vi "iterate_current_block_offset.vi"(8 "error in (no error)":errorcluster, 11 "GenericWriteSignals in":refnum<class "GenericSignalWriter.lvclass">) -> (0 "error out":errorcluster, 2 "finished?":bool, 3 "GenericWriteSignals out":refnum<class "GenericSignalWriter.lvclass">)   [LabVIEW 2010, in "GenericSignalWriter.lvclass"]
uses:
  GenericSignalWriter.lvclass
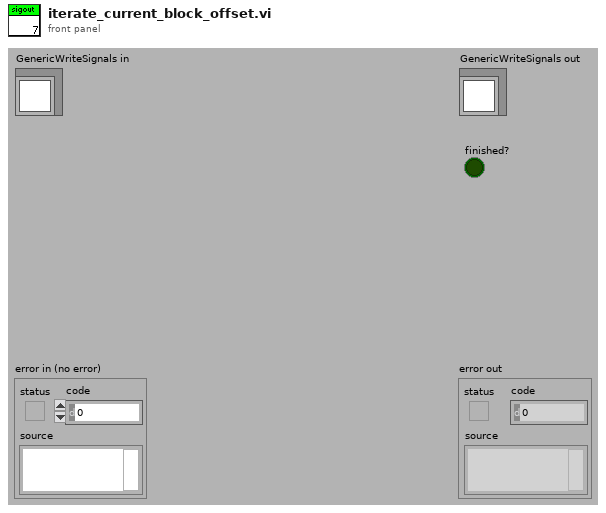
[diagram p1: front panel]
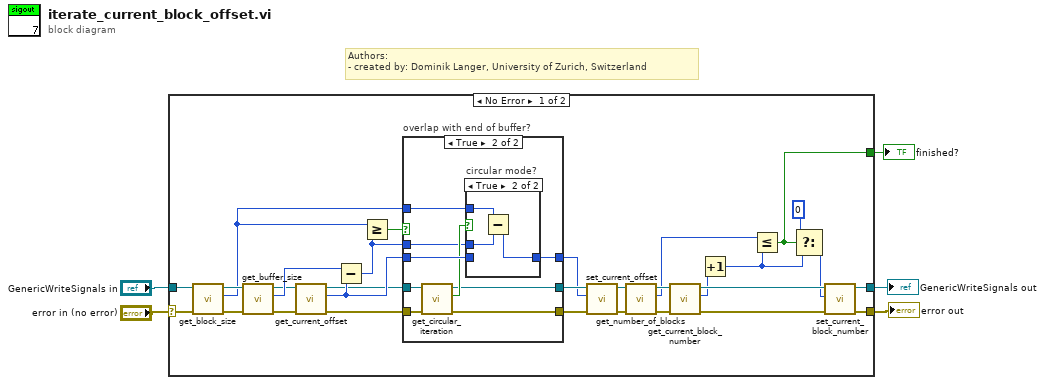
[diagram p0: block diagram]
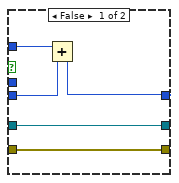
[diagram p2: hidden frame]
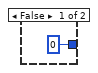
[diagram p3: hidden frame]
diagram:
  # "Authors: \n- created by: Dominik Langer, University of Zurich, Switzerland"
  n1 = case shown="No Error" "error in (no error)" {
    selector: "error in (no error)" -> [w27 w55]
    tunnel: [w18 w55] -> w4
    tunnel: [w19 w54] -> w2
    tunnel: "GenericWriteSignals in" -> [w26 w54]
    tunnel: [w10 _] -> w1
    frame No Error {
      n2 = call "get_block_size.vi"("error in (no error)"=w27, "GenericWriteSignals.lvclass in"=w26) -> ("error out"=w33:errorcluster, "block size"=w29:i32, "GenericWriteSignals.lvclass out"=w32:refnum<class "GenericSignalWriter.lvclass">)  [unwired: 7 out]
      n3 = call-dynamic "get_buffer_size.vi"("error in (no error)"=w33, "GenericWriteSignals.lvclass in"=w32) -> ("error out"=w34:errorcluster, "buffer size (samples)"=w35:i32, "GenericWriteSignals.lvclass out"=w31:refnum<class "GenericSignalWriter.lvclass">)  [unwired: 7 out]
      n4 = call-dynamic "get_current_offset.vi"("error in (no error)"=w34, "GenericWriteSignals.lvclass in"=w31) -> ("error out"=w25:errorcluster, "current offset (samples)"=w28:i32, "GenericWriteSignals.lvclass out"=w24:refnum<class "GenericSignalWriter.lvclass">)  [unwired: 7 out]
      n5 = Subtract(x=w35, y=w28) -> (x-y=w21:i32)
      n6 = Greater Or Equal?(x=w29, y=w21) -> (x >= y?=w30:bool)
      n7 = case "overlap with end of buffer?" shown="True" w30 {
        tunnel: w29 -> [w38 w49]
        tunnel: [w36 w47] -> w20
        tunnel: w28 -> [w37 w48]
        tunnel: w25 -> [w39 w46]
        tunnel: w24 -> [w40 w45]
        tunnel: [w39 w43] -> w23
        tunnel: [w40 w42] -> w22
        tunnel: w21 -> [_ w41]
        frame False {
          n8 = Add(x=w38, y=w37) -> (x+y=w36:i32)
        }
        frame True {
          n9 = call-dynamic "get_circular_iteration.vi"("error in (no error)"=w46, "GenericWriteSignals.lvclass in"=w45) -> ("error out"=w43:errorcluster, "circular iteration?"=w44:bool, "GenericWriteSignals.lvclass out"=w42:refnum<class "GenericSignalWriter.lvclass">)  [unwired: 7 out]
          n10 = case "circular mode?" shown="True" w44 {
            tunnel: w49 -> [_ w53]
            tunnel: w48 -> [_ _]
            tunnel: [0 w51] -> w47
            tunnel: w41 -> [_ w52]
            frame False {
            }
            frame True {
              n11 = Subtract(x=w53, y=w52) -> (x-y=w51:i32)
            }
          }
        }
      }
      n12 = call-dynamic "set_current_offset.vi"("error in (no error)"=w23, "current offset (samples)"=w20, "GenericWriteSignals.lvclass in"=w22) -> ("error out"=w15:errorcluster, "GenericWriteSignals.lvclass out"=w14:refnum<class "GenericSignalWriter.lvclass">)  [unwired: 7 out]
      n13 = call-dynamic "get_number_of_blocks.vi"("error in (no error)"=w15, "GenericWriteSignals in"=w14) -> ("error out"=w13:errorcluster, "number of blocks"=w11:i32, "GenericWriteSignals out"=w12:refnum<class "GenericSignalWriter.lvclass">)  [unwired: 7 out]
      n14 = call-dynamic "get_current_block_number.vi"("error in (no error)"=w13, "GenericWriteSignals.lvclass in"=w12) -> ("error out"=w16:errorcluster, "current block number"=w7:i32, "GenericWriteSignals.lvclass out"=w17:refnum<class "GenericSignalWriter.lvclass">)  [unwired: 7 out]
      n15 = Increment(x=w7) -> (x+1=w6:i32)
      n16 = Less Or Equal?(x=w11, y=w6) -> (x <= y?=w10:bool)
      n17 = Select(t=0, s=w10, f=w6) -> (s? t:f=w8:i32)
      n18 = call-dynamic "set_current_block_number.vi"("error in (no error)"=w16, "current block number"=w8, "GenericWriteSignals.lvclass in"=w17) -> ("error out"=w18:errorcluster, "GenericWriteSignals.lvclass out"=w19:refnum<class "GenericSignalWriter.lvclass">)  [unwired: 7 out]
    }
    frame Error {
    }
  }
  "error out" <- w4
  "GenericWriteSignals out" <- w2
  "finished?" <- w1
